vi "Manage Save Data.vi"(7 "Bench Type":T1, 8 "entrée d'erreur (pas d'erreur)":errorcluster, 9 "Strings []":string[](array[string]), 10 "Property:Tab Test Result":T4(array[cluster]), 11 "Firebase Altyor en entrée":refnum<class "Firebase Altyor.lvclass">) -> (0 "sortie d'erreur":errorcluster, 3 "Firebase Altyor en sortie":refnum<class "Firebase Altyor.lvclass">)   [LabVIEW 2020, in "Library Core.lvlib" / "Actor Test Firebase.lvclass"]
uses:
  Actor Test Firebase.lvclass
  Firebase/Source/Firebase Altyor/Firebase Altyor.lvclass
  C:/Users/ngarcin/OneDrive - Altyor/Standard TB/Class/Firebase/Source/Firebase Driver/Firebase Driver.lvclass
  Commun VI/TypeDef/Commande Test/Commande Value Type.ctl
  Commun VI/TypeDef/Commande Test/Commande Type Test.ctl
  Commun VI/TypeDef/Bench Type.ctl
  Firebase/Source/Firebase AssembledProducts/Firebase AssembledProducts_String/Firebase AssembledProducts_String.lvclass
  Firebase/Source/Firebase PCBA/Firebase Benches_String/Firebase Benches_String.lvclass
  Firebase/Source/Firebase AssembledProducts/Firebase AssembledProducts_Booleen/Firebase AssembledProducts_Booleen.lvclass
  Firebase/Source/Firebase PCBA/Firebase Benches_Booleen/Firebase Benches_Booleen.lvclass
  Firebase/Source/Firebase AssembledProducts/Firebase AssembledProducts_Number/Firebase AssembledProducts_Number.lvclass
  Firebase/Source/Firebase PCBA/Dossier Firebase Benches_Number/Firebase Benches_Number.lvclass
  Actor Test Firebase.lvclass/Actor Test Firebase.ctl
  Commun VI/Library Commun.lvlib
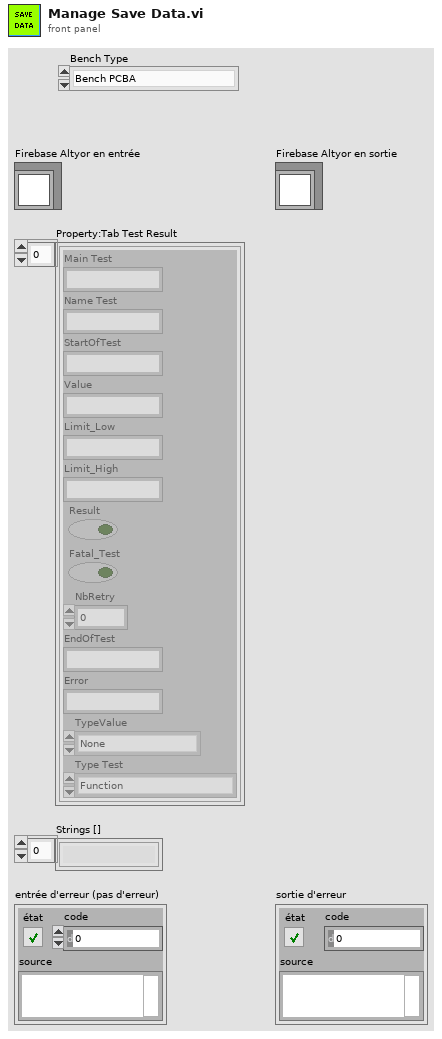
[diagram p1: front panel]
types:
  T1 = typedef "Library Commun.lvlib/Bench Type.ctl" = enum16{"Bench PCBA", "Bench Camera", "Bench Assembly", "Bench PCBA P2193"}
  T2 = typedef "Library Commun.lvlib/Commande Value Type.ctl" = enum16{"None", "String", "Number", "Timestamp", "Boolean", "Array"}
  T3 = typedef "Library Commun.lvlib/Commande Type Test.ctl" = enum16{"Function", "Test", "Calculation"}
  T4 = cluster{"Main Test":string, "Name Test":string, "StartOfTest":string, "Value":string, "Limit_Low":string, "Limit_High":string, "Result":bool, "Fatal_Test":bool, "NbRetry":dbl, "EndOfTest":string, "Error":string, "TypeValue":T2, "Type Test":T3}[]
  T5 = cluster{"Result":cluster{"booleanValue":bool}, "Name":cluster{"stringValue":string}, "StartOfTest":cluster{"timestampValue":string}, "EndOfTest":cluster{"timestampValue":string}, "limit":cluster{"mapValue":cluster{"fields":cluster{"Lower":cluster{"stringValue":string}, "Upper":cluster{"stringValue":string}}}}, "Value":cluster{"stringValue":string}, "Type":cluster{"stringValue":string}, "MainTest":cluster{"stringValue":string}}
  T6 = cluster{"Result":cluster{"booleanValue":bool}, "Name":cluster{"stringValue":string}, "StartOfTest":cluster{"timestampValue":string}, "EndOfTest":cluster{"timestampValue":string}, "limit":cluster{"mapValue":cluster{"fields":cluster{"Lower":cluster{"stringValue":string}, "Upper":cluster{"stringValue":string}}}}, "Value":cluster{"booleanValue":bool}, "Type":cluster{"stringValue":string}, "MainTest":cluster{"stringValue":string}}
  T7 = cluster{"Result":cluster{"booleanValue":bool}, "Name":cluster{"stringValue":string}, "StartOfTest":cluster{"timestampValue":string}, "EndOfTest":cluster{"timestampValue":string}, "limit":cluster{"mapValue":cluster{"fields":cluster{"Lower":cluster{"stringValue":string}, "Upper":cluster{"stringValue":string}}}}, "Value":cluster{"doubleValue":dbl}, "Type":cluster{"stringValue":string}, "MainTest":cluster{"stringValue":string}}
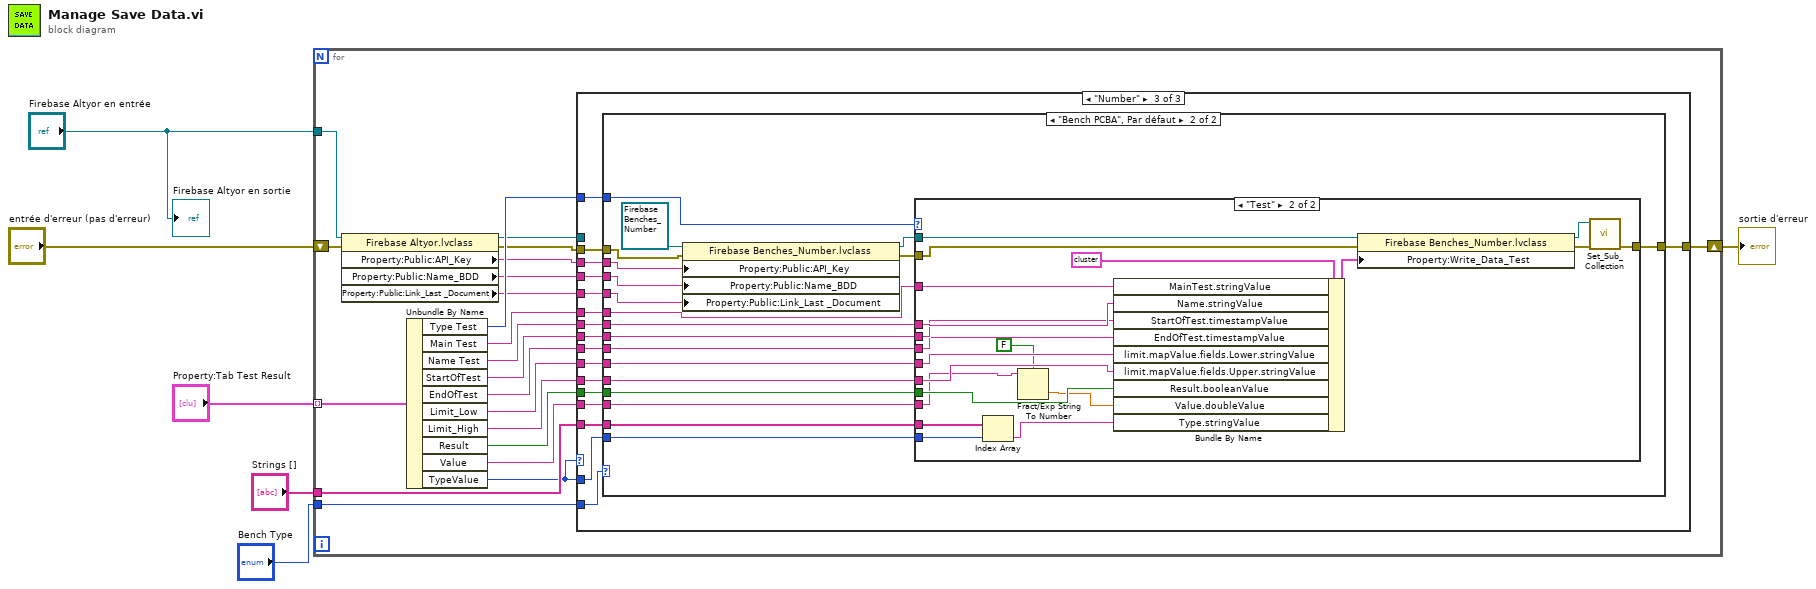
[diagram p0: block diagram]
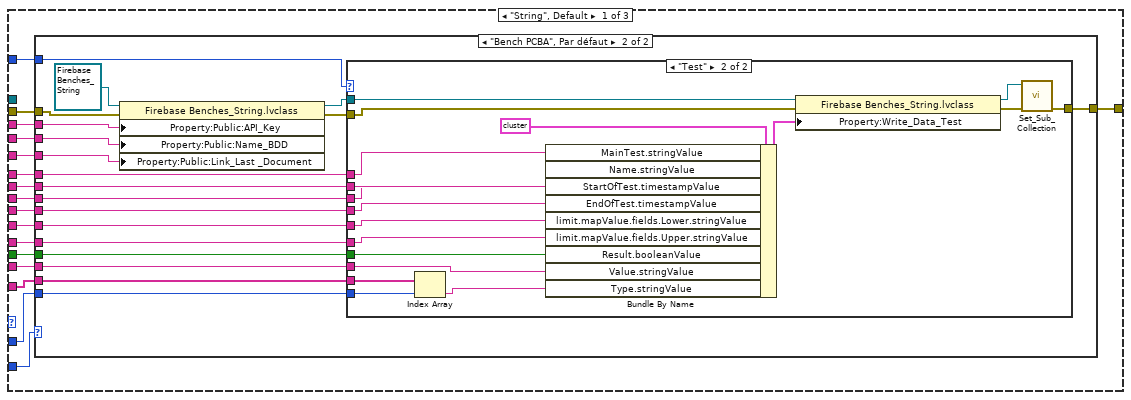
[diagram p2: hidden frame]
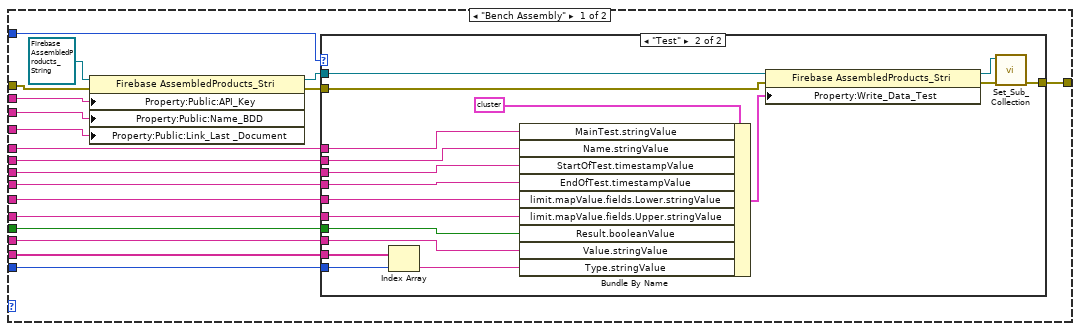
[diagram p3: hidden frame]
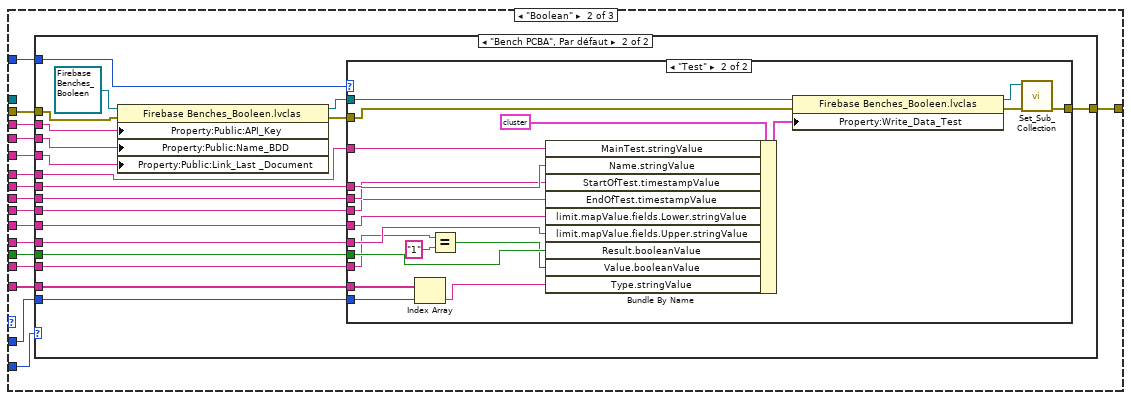
[diagram p6: hidden frame]
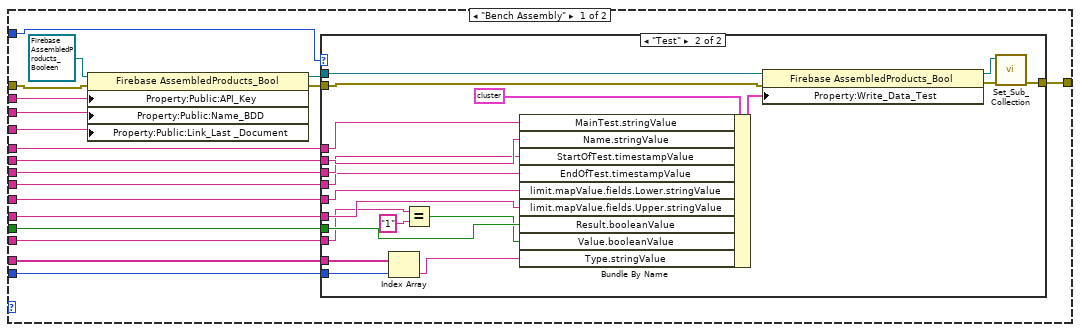
[diagram p7: hidden frame]
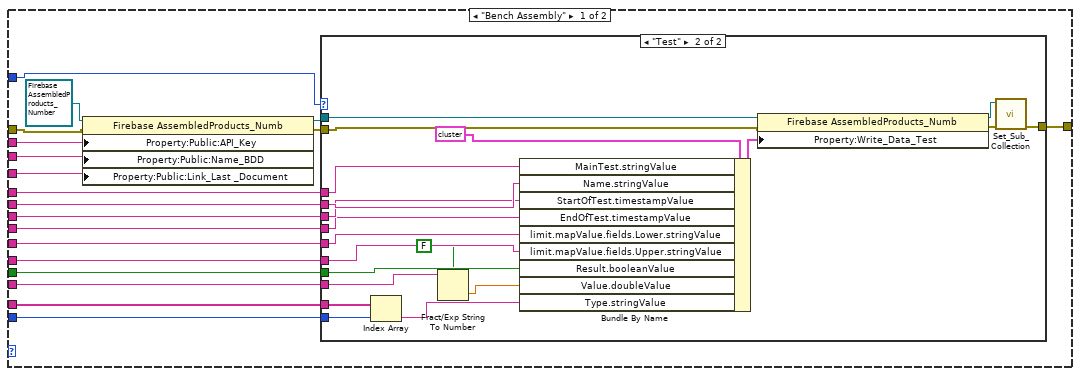
[diagram p10: hidden frame]
diagram:
  n1 = for {
    shift-right: [w27] -> w3
    shift-left: "entrée d'erreur (pas d'erreur)" -> [w10]
    tunnel: "Property:Tab Test Result" -> [w26] mode=indexing
    tunnel: "Strings []" -> [w25]
    tunnel: "Firebase Altyor en entrée" -> [w14]
    tunnel: "Bench Type" -> [w7]
    n2 = property class="Firebase Altyor.lvclass"(reference=w14, error in=w10) -> (reference out=w9:refnum<class "Firebase Altyor.lvclass">, error out=w11:errorcluster, "Property:Public:API_Key"=w13:string, "Property:Public:Name_BDD"=w12:string, "Property:Public:Link_Last _Document"=w8:string)
    n3 = Unbundle By Name(w26) -> ("Type Test"=w16:T3, "Main Test"=w24:string, "Name Test"=w23:string, "StartOfTest"=w22:string, "EndOfTest"=w21:string, "Limit_Low"=w20:string, "Limit_High"=w19:string, "Result"=w18:bool, "Value"=w17:string, "TypeValue"=w15:T2)
    n4 = case shown="\"Number\"" w15 {
      tunnel: [w44 w137 w234] -> w27
      tunnel: w25 -> [w43 w136 w233]
      tunnel: w24 -> [w42 w135 w232]
      tunnel: w23 -> [w41 w134 w231]
      tunnel: w22 -> [w40 w133 w230]
      tunnel: w21 -> [w39 w132 w229]
      tunnel: w20 -> [w38 w131 w228]
      tunnel: w19 -> [w37 w130 w227]
      tunnel: w18 -> [w36 w129 w226]
      tunnel: w17 -> [w35 w128 w225]
      tunnel: w15 -> [w34 w127 w224]
      tunnel: w16 -> [w33 w126 w223]
      tunnel: w13 -> [w31 w125 w222]
      tunnel: w12 -> [w30 w124 w221]
      tunnel: w11 -> [w32 w123 w220]
      tunnel: w9 -> [_ _ _]
      tunnel: w8 -> [w29 w122 w219]
      tunnel: w7 -> [w28 w121 w218]
      frame "String", Default {
        n5 = case shown="\"Bench PCBA\", Par défaut" w28 {
          tunnel: [w63 w101] -> w44
          tunnel: w43 -> [w62 w100]
          tunnel: w42 -> [w61 w99]
          tunnel: w41 -> [w60 w98]
          tunnel: w40 -> [w59 w97]
          tunnel: w39 -> [w58 w96]
          tunnel: w38 -> [w57 w95]
          tunnel: w37 -> [w56 w94]
          tunnel: w36 -> [w55 w93]
          tunnel: w35 -> [w54 w92]
          tunnel: w34 -> [w53 w91]
          tunnel: w33 -> [w52 w90]
          tunnel: w32 -> [w49 w87]
          tunnel: w31 -> [w48 w86]
          tunnel: w30 -> [w47 w85]
          tunnel: w29 -> [w45 w84]
          frame "Bench Assembly" {
            n6 = property class="Firebase AssembledProducts_Stri"(reference=refnum<class "Firebase AssembledProducts_String.lvclass"> refnum ("Library FireBase.lvlib:Firebase AssembledProducts_String.lvclass"), error in=w49, "Property:Public:API_Key"=w48, "Property:Public:Name_BDD"=w47, "Property:Public:Link_Last _Document"=w45) -> (reference out=w50:refnum<class "Firebase AssembledProducts_String.lvclass">, error out=w51:errorcluster)
            n7 = case shown="\"Test\"" w52 {
              tunnel: w50 -> [_ w82]
              tunnel: w51 -> [w64 w81]
              tunnel: [w64 w79] -> w63
              tunnel: w62 -> [_ w75]
              tunnel: w61 -> [_ w73]
              tunnel: w60 -> [_ w72]
              tunnel: w59 -> [_ w71]
              tunnel: w58 -> [_ w70]
              tunnel: w57 -> [_ w69]
              tunnel: w56 -> [_ w68]
              tunnel: w55 -> [_ w67]
              tunnel: w54 -> [_ w66]
              tunnel: w53 -> [_ w65]
              frame Default {
              }
              frame "Test" {
                n8 = Index Array(array=w75, index=w65) -> (element=w74:string)
                n9 = Bundle By Name(cluster=T5 {"Result"={"booleanValue"=FALSE}, "Name"={"stringValue"=""}, "StartOfTest"={"timestampValue"=""}, "EndOfTest"={"timestampValue"=""}, "limit"={"mapValue"={"fields"={"Lower"={"stringValue"=""}, "Upper"={"stringValue"=""}}}}, "Value"={"stringValue"=""}, "Type"={"stringValue"=""}, "MainTest"={"stringValue"=""}} ("Write_Data_Test"), "MainTest.stringValue"=w73, "Name.stringValue"=w72, "StartOfTest.timestampValue"=w71, "EndOfTest.timestampValue"=w70, "limit.mapValue.fields.Lower.stringValue"=w69, "limit.mapValue.fields.Upper.stringValue"=w68, "Result.booleanValue"=w67, "Value.stringValue"=w66, "Type.stringValue"=w74) -> (w76:T5)
                n10 = property class="Firebase AssembledProducts_Stri"(reference=w82, error in=w81, "Property:Write_Data_Test"=w76) -> (reference out=w78:refnum<class "Firebase AssembledProducts_String.lvclass">, error out=w80:errorcluster)
                n11 = call-dynamic "Set_Sub_Collection.vi"("error in (no error)"=w80, "Firebase PCBA en entrée"=w78) -> ("error out"=w79:errorcluster)  [unwired: 8 in, 1 out]
              }
            }
          }
          frame "Bench PCBA", Default {
            n12 = property class="Firebase Benches_String.lvclass"(reference=refnum<class "Firebase Benches_String.lvclass"> refnum ("Library FireBase.lvlib:Firebase Benches_String.lvclass"), error in=w87, "Property:Public:API_Key"=w86, "Property:Public:Name_BDD"=w85, "Property:Public:Link_Last _Document"=w84) -> (reference out=w88:refnum<class "Firebase Benches_String.lvclass">, error out=w89:errorcluster)
            n13 = case shown="\"Test\"" w90 {
              tunnel: w88 -> [_ w120]
              tunnel: w89 -> [w102 w119]
              tunnel: [w102 w117] -> w101
              tunnel: w100 -> [_ w113]
              tunnel: w99 -> [_ w111]
              tunnel: w98 -> [_ w110]
              tunnel: w97 -> [_ w109]
              tunnel: w96 -> [_ w108]
              tunnel: w95 -> [_ w107]
              tunnel: w94 -> [_ w106]
              tunnel: w93 -> [_ w105]
              tunnel: w92 -> [_ w104]
              tunnel: w91 -> [_ w103]
              frame Default {
              }
              frame "Test" {
                n14 = Index Array(array=w113, index=w103) -> (element=w112:string)
                n15 = Bundle By Name(cluster=T5 {"Result"={"booleanValue"=FALSE}, "Name"={"stringValue"=""}, "StartOfTest"={"timestampValue"=""}, "EndOfTest"={"timestampValue"=""}, "limit"={"mapValue"={"fields"={"Lower"={"stringValue"=""}, "Upper"={"stringValue"=""}}}}, "Value"={"stringValue"=""}, "Type"={"stringValue"=""}, "MainTest"={"stringValue"=""}} ("Write_Data_Test"), "MainTest.stringValue"=w111, "Name.stringValue"=w110, "StartOfTest.timestampValue"=w109, "EndOfTest.timestampValue"=w108, "limit.mapValue.fields.Lower.stringValue"=w107, "limit.mapValue.fields.Upper.stringValue"=w106, "Result.booleanValue"=w105, "Value.stringValue"=w104, "Type.stringValue"=w112) -> (w114:T5)
                n16 = property class="Firebase Benches_String.lvclass"(reference=w120, error in=w119, "Property:Write_Data_Test"=w114) -> (reference out=w116:refnum<class "Firebase Benches_String.lvclass">, error out=w118:errorcluster)
                n17 = call-dynamic "Set_Sub_Collection.vi"("error in (no error)"=w118, "Firebase PCBA en entrée"=w116) -> ("error out"=w117:errorcluster)  [unwired: 8 in, 1 out]
              }
            }
          }
        }
      }
      frame "Boolean" {
        n18 = case shown="\"Bench PCBA\", Par défaut" w121 {
          tunnel: [w156 w196] -> w137
          tunnel: w136 -> [w155 w195]
          tunnel: w135 -> [w154 w194]
          tunnel: w134 -> [w153 w193]
          tunnel: w133 -> [w152 w192]
          tunnel: w132 -> [w151 w191]
          tunnel: w131 -> [w150 w190]
          tunnel: w130 -> [w149 w189]
          tunnel: w129 -> [w148 w188]
          tunnel: w128 -> [w147 w187]
          tunnel: w127 -> [w146 w186]
          tunnel: w126 -> [w145 w185]
          tunnel: w125 -> [w143 w184]
          tunnel: w124 -> [w142 w183]
          tunnel: w123 -> [w141 w182]
          tunnel: w122 -> [w138 w179]
          frame "Bench Assembly" {
            n19 = property class="Firebase AssembledProducts_Bool"(reference=refnum<class "Firebase AssembledProducts_Booleen.lvclass"> refnum ("Library FireBase.lvlib:Firebase AssembledProducts_Booleen.lvclass"), error in=w141, "Property:Public:API_Key"=w143, "Property:Public:Name_BDD"=w142, "Property:Public:Link_Last _Document"=w138) -> (reference out=w140:refnum<class "Firebase AssembledProducts_Booleen.lvclass">, error out=w139:errorcluster)
            n20 = case shown="\"Test\"" w145 {
              tunnel: [w157 w176] -> w156
              tunnel: w155 -> [_ w174]
              tunnel: w154 -> [_ w172]
              tunnel: w153 -> [_ w171]
              tunnel: w152 -> [_ w170]
              tunnel: w151 -> [_ w169]
              tunnel: w150 -> [_ w168]
              tunnel: w149 -> [_ w167]
              tunnel: w148 -> [_ w166]
              tunnel: w147 -> [_ w165]
              tunnel: w146 -> [_ w164]
              tunnel: w140 -> [_ w159]
              tunnel: w139 -> [w157 w158]
              frame Default {
              }
              frame "Test" {
                n21 = Index Array(array=w174, index=w164) -> (element=w173:string)
                n22 = Equal?(x=w165, y="1") -> (x = y?=w162:bool)
                n23 = Bundle By Name(cluster=T6 {"Result"={"booleanValue"=FALSE}, "Name"={"stringValue"=""}, "StartOfTest"={"timestampValue"=""}, "EndOfTest"={"timestampValue"=""}, "limit"={"mapValue"={"fields"={"Lower"={"stringValue"=""}, "Upper"={"stringValue"=""}}}}, "Value"={"booleanValue"=FALSE}, "Type"={"stringValue"=""}, "MainTest"={"stringValue"=""}} ("Write_Data_Test"), "MainTest.stringValue"=w172, "Name.stringValue"=w171, "StartOfTest.timestampValue"=w170, "EndOfTest.timestampValue"=w169, "limit.mapValue.fields.Lower.stringValue"=w168, "limit.mapValue.fields.Upper.stringValue"=w167, "Result.booleanValue"=w166, "Value.booleanValue"=w162, "Type.stringValue"=w173) -> (w160:T6)
                n24 = property class="Firebase AssembledProducts_Bool"(reference=w159, error in=w158, "Property:Write_Data_Test"=w160) -> (reference out=w175:refnum<class "Firebase AssembledProducts_Booleen.lvclass">, error out=w177:errorcluster)
                n25 = call-dynamic "Set_Sub_Collection.vi"("error in (no error)"=w177, "Firebase PCBA en entrée"=w175) -> ("error out"=w176:errorcluster)  [unwired: 8 in, 1 out]
              }
            }
          }
          frame "Bench PCBA", Default {
            n26 = property class="Firebase Benches_Booleen.lvclas"(reference=refnum<class "Firebase Benches_Booleen.lvclass"> refnum ("Library FireBase.lvlib:Firebase Benches_Booleen.lvclass"), error in=w182, "Property:Public:API_Key"=w184, "Property:Public:Name_BDD"=w183, "Property:Public:Link_Last _Document"=w179) -> (reference out=w181:refnum<class "Firebase Benches_Booleen.lvclass">, error out=w180:errorcluster)
            n27 = case shown="\"Test\"" w185 {
              tunnel: [w197 w216] -> w196
              tunnel: w195 -> [_ w214]
              tunnel: w194 -> [_ w212]
              tunnel: w193 -> [_ w211]
              tunnel: w192 -> [_ w210]
              tunnel: w191 -> [_ w209]
              tunnel: w190 -> [_ w208]
              tunnel: w189 -> [_ w207]
              tunnel: w188 -> [_ w206]
              tunnel: w187 -> [_ w205]
              tunnel: w186 -> [_ w204]
              tunnel: w181 -> [_ w199]
              tunnel: w180 -> [w197 w198]
              frame Default {
              }
              frame "Test" {
                n28 = Index Array(array=w214, index=w204) -> (element=w213:string)
                n29 = Equal?(x=w205, y="1") -> (x = y?=w202:bool)
                n30 = Bundle By Name(cluster=T6 {"Result"={"booleanValue"=FALSE}, "Name"={"stringValue"=""}, "StartOfTest"={"timestampValue"=""}, "EndOfTest"={"timestampValue"=""}, "limit"={"mapValue"={"fields"={"Lower"={"stringValue"=""}, "Upper"={"stringValue"=""}}}}, "Value"={"booleanValue"=FALSE}, "Type"={"stringValue"=""}, "MainTest"={"stringValue"=""}} ("Write_Data_Test"), "MainTest.stringValue"=w212, "Name.stringValue"=w211, "StartOfTest.timestampValue"=w210, "EndOfTest.timestampValue"=w209, "limit.mapValue.fields.Lower.stringValue"=w208, "limit.mapValue.fields.Upper.stringValue"=w207, "Result.booleanValue"=w206, "Value.booleanValue"=w202, "Type.stringValue"=w213) -> (w200:T6)
                n31 = property class="Firebase Benches_Booleen.lvclas"(reference=w199, error in=w198, "Property:Write_Data_Test"=w200) -> (reference out=w215:refnum<class "Firebase Benches_Booleen.lvclass">, error out=w217:errorcluster)
                n32 = call-dynamic "Set_Sub_Collection.vi"("error in (no error)"=w217, "Firebase PCBA en entrée"=w215) -> ("error out"=w216:errorcluster)  [unwired: 8 in, 1 out]
              }
            }
          }
        }
      }
      frame "Number" {
        n33 = case shown="\"Bench PCBA\", Par défaut" w218 {
          tunnel: [w253 w293] -> w234
          tunnel: w233 -> [w252 w292]
          tunnel: w232 -> [w251 w291]
          tunnel: w231 -> [w250 w290]
          tunnel: w230 -> [w249 w289]
          tunnel: w229 -> [w248 w288]
          tunnel: w228 -> [w247 w287]
          tunnel: w227 -> [w246 w286]
          tunnel: w226 -> [w245 w285]
          tunnel: w225 -> [w244 w284]
          tunnel: w224 -> [w243 w283]
          tunnel: w223 -> [w242 w282]
          tunnel: w222 -> [w241 w281]
          tunnel: w221 -> [w240 w280]
          tunnel: w220 -> [w239 w279]
          tunnel: w219 -> [w236 w276]
          frame "Bench Assembly" {
            n34 = property class="Firebase AssembledProducts_Numb"(reference=refnum<class "Firebase AssembledProducts_Number.lvclass"> refnum ("Library FireBase.lvlib:Firebase AssembledProducts_Number.lvclass"), error in=w239, "Property:Public:API_Key"=w241, "Property:Public:Name_BDD"=w240, "Property:Public:Link_Last _Document"=w236) -> (reference out=w238:refnum<class "Firebase AssembledProducts_Number.lvclass">, error out=w237:errorcluster)
            n35 = case shown="\"Test\"" w242 {
              tunnel: [w254 w273] -> w253
              tunnel: w252 -> [_ w271]
              tunnel: w251 -> [_ w269]
              tunnel: w250 -> [_ w268]
              tunnel: w249 -> [_ w267]
              tunnel: w248 -> [_ w266]
              tunnel: w247 -> [_ w265]
              tunnel: w246 -> [_ w264]
              tunnel: w245 -> [_ w263]
              tunnel: w244 -> [_ w257]
              tunnel: w243 -> [_ w262]
              tunnel: w238 -> [_ w260]
              tunnel: w237 -> [w254 w259]
              frame Default {
              }
              frame "Test" {
                n36 = Index Array(array=w271, index=w262) -> (element=w270:string)
                n37 = Fract/Exp String To Number(use system decimal point (T)=FALSE ("utiliser le séparateur décimal du système (V)"), string=w257) -> (number=w256:dbl)  [unwired: 2 in, 1 out]
                n38 = Bundle By Name(cluster=T7 {"Result"={"booleanValue"=FALSE}, "Name"={"stringValue"=""}, "StartOfTest"={"timestampValue"=""}, "EndOfTest"={"timestampValue"=""}, "limit"={"mapValue"={"fields"={"Lower"={"stringValue"=""}, "Upper"={"stringValue"=""}}}}, "Value"={"doubleValue"=0.0}, "Type"={"stringValue"=""}, "MainTest"={"stringValue"=""}} ("Write_Data_Test"), "MainTest.stringValue"=w269, "Name.stringValue"=w268, "StartOfTest.timestampValue"=w267, "EndOfTest.timestampValue"=w266, "limit.mapValue.fields.Lower.stringValue"=w265, "limit.mapValue.fields.Upper.stringValue"=w264, "Result.booleanValue"=w263, "Value.doubleValue"=w256, "Type.stringValue"=w270) -> (w261:T7)
                n39 = property class="Firebase AssembledProducts_Numb"(reference=w260, error in=w259, "Property:Write_Data_Test"=w261) -> (reference out=w272:refnum<class "Firebase AssembledProducts_Number.lvclass">, error out=w274:errorcluster)
                n40 = call-dynamic "Set_Sub_Collection.vi"("error in (no error)"=w274, "Firebase PCBA en entrée"=w272) -> ("error out"=w273:errorcluster)  [unwired: 8 in, 1 out]
              }
            }
          }
          frame "Bench PCBA", Default {
            n41 = property class="Firebase Benches_Number.lvclass"(reference=refnum<class "Firebase Benches_Number.lvclass"> refnum ("Library FireBase.lvlib:Firebase Benches_Number.lvclass"), error in=w279, "Property:Public:API_Key"=w281, "Property:Public:Name_BDD"=w280, "Property:Public:Link_Last _Document"=w276) -> (reference out=w278:refnum<class "Firebase Benches_Number.lvclass">, error out=w277:errorcluster)
            n42 = case shown="\"Test\"" w282 {
              tunnel: [w294 w313] -> w293
              tunnel: w292 -> [_ w311]
              tunnel: w291 -> [_ w309]
              tunnel: w290 -> [_ w308]
              tunnel: w289 -> [_ w307]
              tunnel: w288 -> [_ w306]
              tunnel: w287 -> [_ w305]
              tunnel: w286 -> [_ w304]
              tunnel: w285 -> [_ w303]
              tunnel: w284 -> [_ w297]
              tunnel: w283 -> [_ w302]
              tunnel: w278 -> [_ w300]
              tunnel: w277 -> [w294 w299]
              frame Default {
              }
              frame "Test" {
                n43 = Index Array(array=w311, index=w302) -> (element=w310:string)
                n44 = Fract/Exp String To Number(use system decimal point (T)=FALSE ("utiliser le séparateur décimal du système (V)"), string=w297) -> (number=w296:dbl)  [unwired: 2 in, 1 out]
                n45 = Bundle By Name(cluster=T7 {"Result"={"booleanValue"=FALSE}, "Name"={"stringValue"=""}, "StartOfTest"={"timestampValue"=""}, "EndOfTest"={"timestampValue"=""}, "limit"={"mapValue"={"fields"={"Lower"={"stringValue"=""}, "Upper"={"stringValue"=""}}}}, "Value"={"doubleValue"=0.0}, "Type"={"stringValue"=""}, "MainTest"={"stringValue"=""}} ("Write_Data_Test"), "MainTest.stringValue"=w309, "Name.stringValue"=w308, "StartOfTest.timestampValue"=w307, "EndOfTest.timestampValue"=w306, "limit.mapValue.fields.Lower.stringValue"=w305, "limit.mapValue.fields.Upper.stringValue"=w304, "Result.booleanValue"=w303, "Value.doubleValue"=w296, "Type.stringValue"=w310) -> (w301:T7)
                n46 = property class="Firebase Benches_Number.lvclass"(reference=w300, error in=w299, "Property:Write_Data_Test"=w301) -> (reference out=w312:refnum<class "Firebase Benches_Number.lvclass">, error out=w314:errorcluster)
                n47 = call-dynamic "Set_Sub_Collection.vi"("error in (no error)"=w314, "Firebase PCBA en entrée"=w312) -> ("error out"=w313:errorcluster)  [unwired: 8 in, 1 out]
              }
            }
          }
        }
      }
    }
  }
  "sortie d'erreur" <- w3
  "Firebase Altyor en sortie" <- "Firebase Altyor en entrée"
